vi "MotionProfileBegin.vi"(8 "error in (no error)":errorcluster) -> (0 "error out":errorcluster)   [LabVIEW 2019, in "Drive.lvlib" / "CTRE Drive.lvclass"]
uses:
  CTRE Drive.lvclass
  <vilib>/Rock Robotics/WPI/ThirdParty/Phoenix-LabVIEW/Motor Controller/Controls/CTRE_Phoenix_MotorControl_MotionProfileTrajectoryPoint.ctl
  <vilib>/Utility/file.llb/Read Delimited Spreadsheet (DBL).vi
  <vilib>/Rock Robotics/WPI/ThirdParty/Phoenix-LabVIEW/Motor Controller/Closed Loop/Motion Profile/CTRE_Phoenix_MotorControl_BufferedTrajectoryPointStream_WriteAll.vi
  <vilib>/Rock Robotics/WPI/ThirdParty/Phoenix-LabVIEW/Motor Controller/Closed Loop/Motion Profile/CTRE_Phoenix_MotorControl_BufferedTrajectoryPointStream_WriteOne.vi
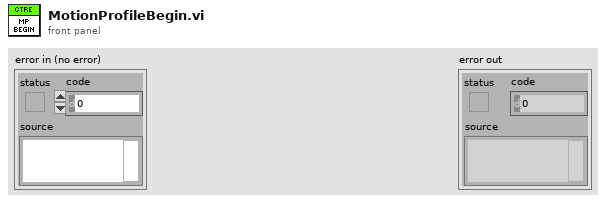
[diagram p1: front panel]
types:
  T1 = typedef "CTRE_Phoenix_MotorControl_MotionProfileTrajectoryPoint.ctl" = cluster{"Position":dbl, "Velocity":dbl, "Arbitrary Feed Forward":dbl, "Auxiliary Position":dbl, "Auxiliary Velocity":dbl, "Auxiliary Arbitrary Feed Forward":dbl, "Profile Slot Select":i32, "Auxiliary Profile Slot Select":i32, "isLastPoint?":bool, "Zero Position?":bool, "durationMs":u32, "Use Aux PID?":bool}
  T2 = typedef "CTRE_Phoenix_MotorControl_BufferedTrajectoryPointStream_DeviceRef.ctl" = cluster{"Handle":u64, "Library Path":path}
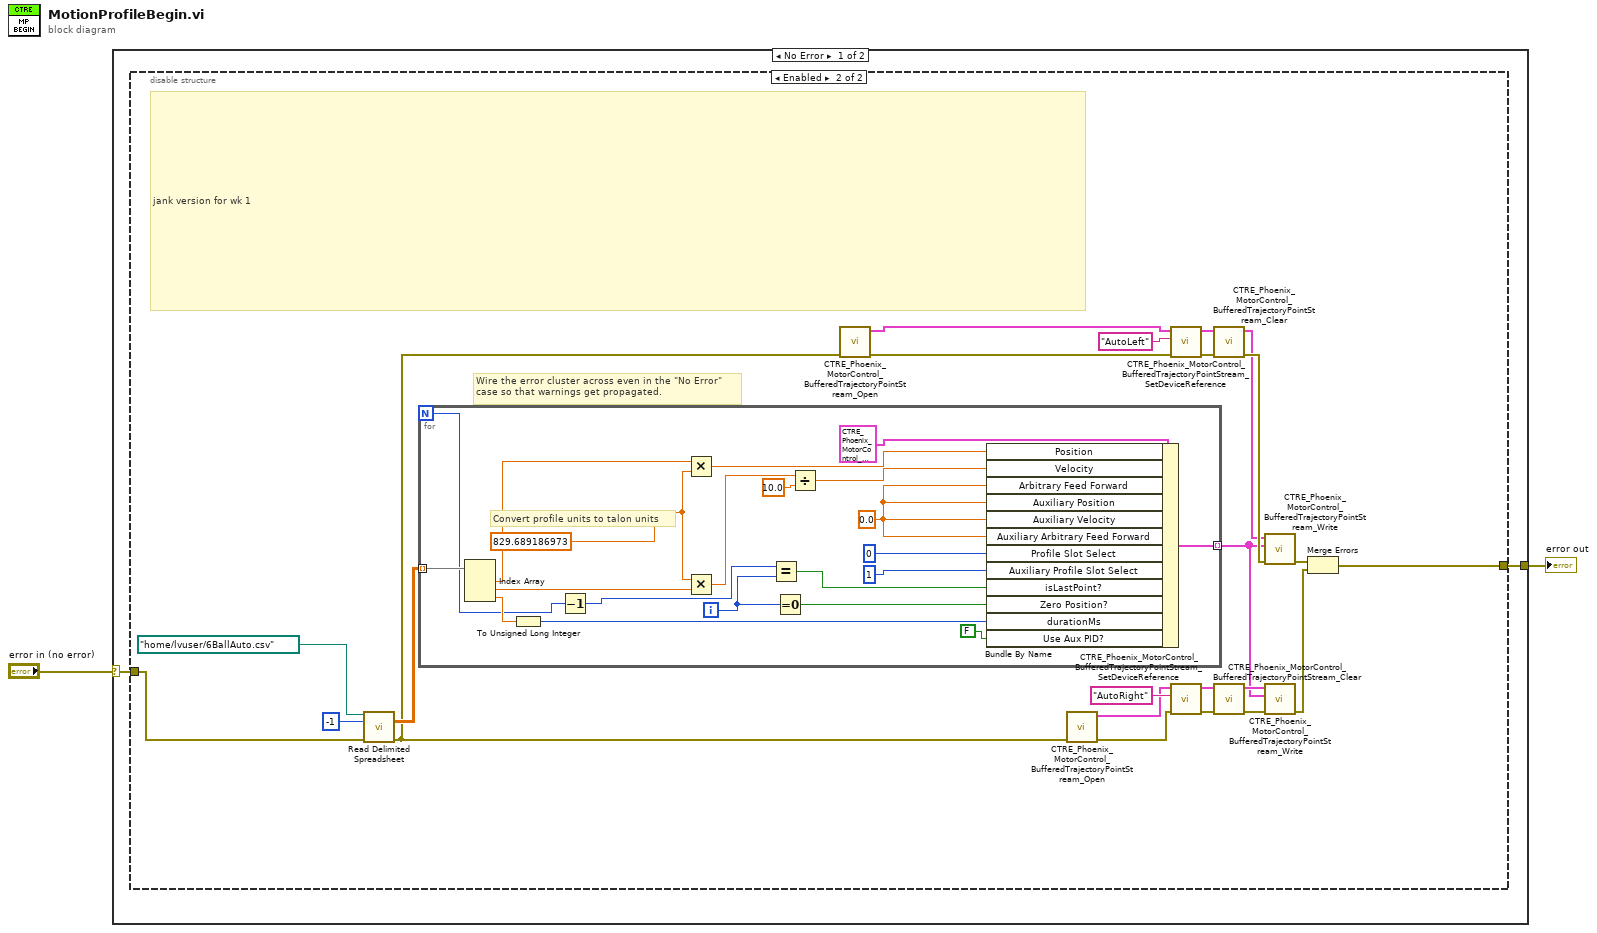
[diagram p0: block diagram]
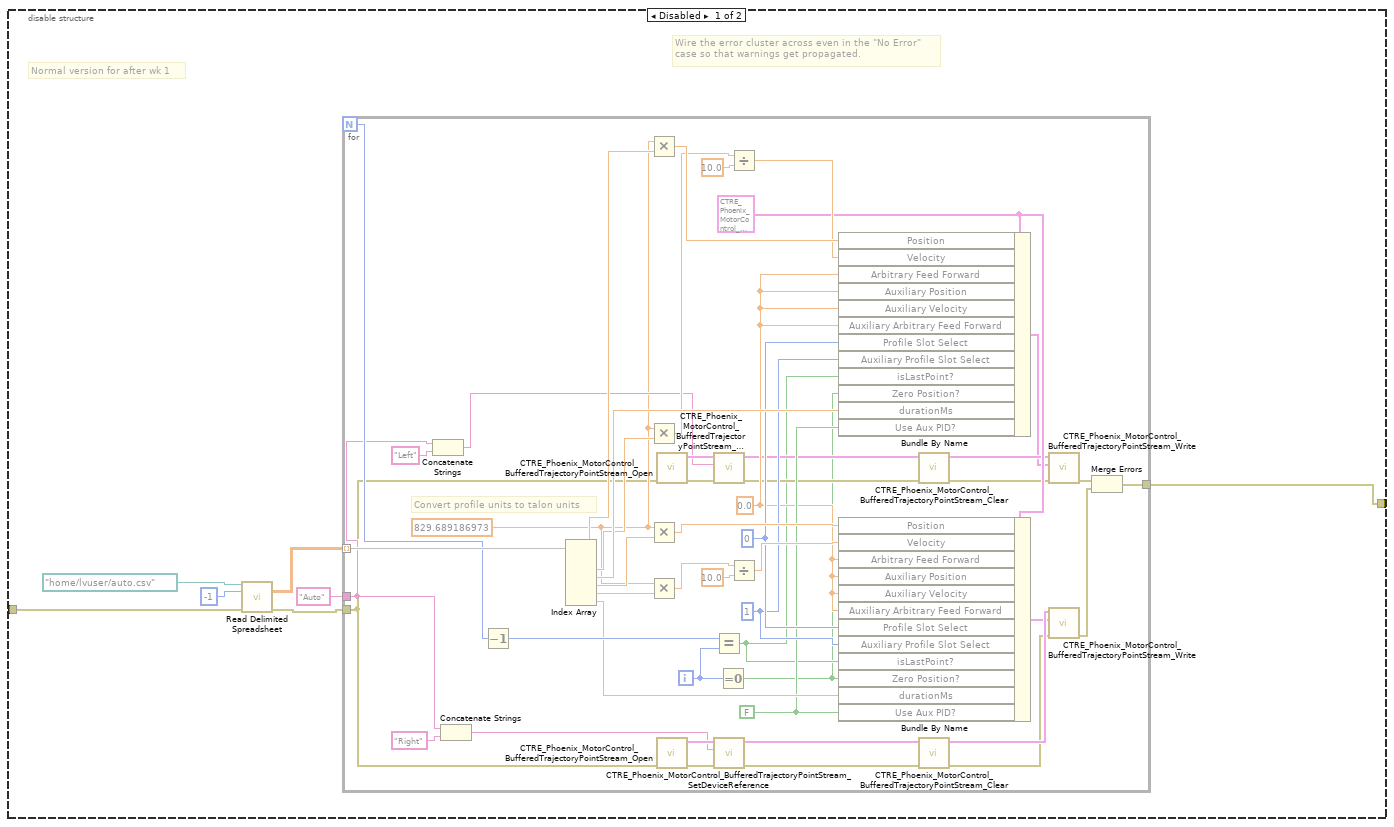
[diagram p2: hidden frame]
diagram:
  n1 = case shown="No Error" "error in (no error)" {
    selector: "error in (no error)" -> [w4 w105]
    tunnel: [w3 w105] -> w1
    frame No Error {
      n2 = disable-structure shown="Enabled" {
        disable-tunnel: w4 -> [w10 w80]
        disable-tunnel: [w9 w63] -> w3
        frame Disabled {
          # "Normal version for after wk 1"
          # "Wire the error cluster across even in the \"No Error\"\ncase so that warnings get propagated."
          n3 = call-poly <vilib>:"Read Delimited Spreadsheet.vi"("file path (dialog if empty)"=path "/home/lvuser/auto.csv" ("file path (use dialog)"), "number of rows (all:-1)"=-1, "error in (no error)"=w10) -> ("all rows"=w8:dbl[][], "error out"=w7:errorcluster)  [unwired: 7 in, 4 out]
          n4 = for {
            N -> [w42]
            tunnel: w8 -> [w52] mode=indexing
            tunnel: "Auto" -> [w30]
            tunnel: w7 -> [w15]
            tunnel: [w12] -> w9
            i -> [w38]
            w18 = 829.689186973 ("x")
            w41 = FALSE ("Use Aux PID?")
            w43 = 1 ("Auxiliary Profile Slot Select")
            w44 = 0 ("Profile Slot Select")
            w39 = 0.0 ("Arbitrary Feed Forward")
            w40 = T1 {"Position"=0.0, "Velocity"=0.0, "Arbitrary Feed Forward"=0.0, "Auxiliary Position"=0.0, "Auxiliary Velocity"=0.0, "Auxiliary Arbitrary Feed Forward"=0.0, "Profile Slot Select"=0, "Auxiliary Profile Slot Select"=0, "isLastPoint?"=FALSE, "Zero Position?"=FALSE, "durationMs"=0, "Use Aux PID?"=FALSE} ("Trajectory Point")
            # "Convert profile units to talon units"
            n5 = Concatenate Strings(w30, "Left" ("string")) -> (w28:string)
            n6 = Concatenate Strings(w30, "Right" ("string")) -> (w27:string)
            n7 = Decrement(x=w42) -> (x-1=w60:i32)
            n8 = Index Array(array=w52) -> (element #1=w58:dbl, element #2=w54:dbl, element #3=w59:dbl, element #4=w49:dbl, element #5=w48:dbl, element #6=w47:dbl)  [unwired: 6 in]
            n9 = Multiply(x=w18, y=w58) -> (x*y=w57:dbl)
            n10 = Multiply(x=w18, y=w54) -> (x*y=w56:dbl)
            n11 = Multiply(x=w18, y=w49) -> (x*y=w46:dbl)
            n12 = Multiply(x=w18, y=w48) -> (x*y=w51:dbl)
            n13 = call <vilib>:"CTRE_Phoenix_MotorControl_BufferedTrajectoryPointStream_Open.vi"("error in"=w15) -> ("error out"=w21:errorcluster, "BufferedTrajectoryPointStream_DevRef"=w32:T2)  [unwired: 9 in]
            n14 = call <vilib>:"CTRE_Phoenix_MotorControl_BufferedTrajectoryPointStream_Open.vi"("error in"=w15) -> ("error out"=w25:errorcluster, "BufferedTrajectoryPointStream_DevRef"=w35:T2)  [unwired: 9 in]
            n15 = call <vilib>:"CTRE_Phoenix_MotorControl_BufferedTrajectoryPointStream_SetDeviceReference.vi"("error in (no error)"=w21, "refnum name"=w28, "BufferedTrajectoryPointStream_DevRef"=w32) -> ("error out"=w22:errorcluster, "BufferedTrajectoryPointStream_DevRef"=w33:T2)  [unwired: 7 in]
            n16 = Equal?(x=w60, y=w38) -> (x = y?=w17:bool)
            n17 = call <vilib>:"CTRE_Phoenix_MotorControl_BufferedTrajectoryPointStream_SetDeviceReference.vi"("error in (no error)"=w25, "refnum name"=w27, "BufferedTrajectoryPointStream_DevRef"=w35) -> ("error out"=w26:errorcluster, "BufferedTrajectoryPointStream_DevRef"=w36:T2)  [unwired: 7 in]
            n18 = Equal To 0?(x=w38) -> (x = 0?=w16:bool)
            n19 = Divide(x=w56, y=10.0) -> (x/y=w53:dbl)
            n20 = Divide(x=w51, y=10.0) -> (x/y=w45:dbl)
            n21 = Bundle By Name(cluster=w40, "Position"=w57, "Velocity"=w53, "Arbitrary Feed Forward"=w39, "Auxiliary Position"=w39, "Auxiliary Velocity"=w39, "Auxiliary Arbitrary Feed Forward"=w39, "Profile Slot Select"=w44, "Auxiliary Profile Slot Select"=w43, "isLastPoint?"=w17, "Zero Position?"=w16, "durationMs"=w59, "Use Aux PID?"=w41) -> (w20:T1)
            n22 = Bundle By Name(cluster=w40, "Position"=w46, "Velocity"=w45, "Arbitrary Feed Forward"=w39, "Auxiliary Position"=w39, "Auxiliary Velocity"=w39, "Auxiliary Arbitrary Feed Forward"=w39, "Profile Slot Select"=w44, "Auxiliary Profile Slot Select"=w43, "isLastPoint?"=w17, "Zero Position?"=w16, "durationMs"=w47, "Use Aux PID?"=w41) -> (w19:T1)
            n23 = call <vilib>:"CTRE_Phoenix_MotorControl_BufferedTrajectoryPointStream_Clear.vi"("error in"=w22, "BufferedTrajectoryPointStream_DevRef"=w33) -> ("error out"=w23:errorcluster, "BufferedTrajectoryPointStream_DevRef"=w34:T2)  [unwired: 8 in]
            n24 = call <vilib>:"CTRE_Phoenix_MotorControl_BufferedTrajectoryPointStream_Clear.vi"("error in"=w26, "BufferedTrajectoryPointStream_DevRef"=w36) -> ("error out"=w24:errorcluster, "BufferedTrajectoryPointStream_DevRef"=w37:T2)  [unwired: 8 in]
            n25 = call-poly <vilib>:"CTRE_Phoenix_MotorControl_BufferedTrajectoryPointStream_Write.vi"("error in"=w23, "Trajectory Point"=w20, "BufferedTrajectoryPointStream_DevRef"=w34) -> ("error out"=w14:errorcluster)  [unwired: 7 in, 1 out]
            n26 = call-poly <vilib>:"CTRE_Phoenix_MotorControl_BufferedTrajectoryPointStream_Write.vi"("error in"=w24, "Trajectory Point"=w19, "BufferedTrajectoryPointStream_DevRef"=w37) -> ("error out"=w13:errorcluster)  [unwired: 7 in, 1 out]
            n27 = Merge Errors(w14, w13) -> (w12:errorcluster)
          }
        }
        frame Enabled {
          # "Wire the error cluster across even in the \"No Error\"\ncase so that warnings get propagated."
          # "jank version for wk 1"
          n28 = call-poly <vilib>:"Read Delimited Spreadsheet.vi"("file path (dialog if empty)"=path "/home/lvuser/6BallAuto.csv" ("file path (use dialog)"), "number of rows (all:-1)"=-1, "error in (no error)"=w80) -> ("all rows"=w82:dbl[][], "error out"=w64:errorcluster)  [unwired: 7 in, 4 out]
          n29 = for {
            N -> [w93]
            tunnel: w82 -> [w96] mode=indexing
            tunnel: [w85] -> w61 mode=indexing
            i -> [w89]
            w84 = 829.689186973 ("x")
            w90 = 0.0 ("Arbitrary Feed Forward")
            # "Convert profile units to talon units"
            n30 = Index Array(array=w96) -> (element #1=w102:dbl, element #2=w98:dbl, element #3=w103:dbl)  [unwired: 3 in]
            n31 = To Unsigned Long Integer(number=w103) -> (unsigned 32bit integer=w86:u32)
            n32 = Decrement(x=w93) -> (x-1=w104:i32)
            n33 = Multiply(x=w102, y=w84) -> (x*y=w101:dbl)
            n34 = Multiply(x=w84, y=w98) -> (x*y=w100:dbl)
            n35 = Equal?(x=w104, y=w89) -> (x = y?=w88:bool)
            n36 = Equal To 0?(x=w89) -> (x = 0?=w87:bool)
            n37 = Divide(x=w100, y=10.0) -> (x/y=w97:dbl)
            n38 = Bundle By Name(cluster=T1 {"Position"=0.0, "Velocity"=0.0, "Arbitrary Feed Forward"=0.0, "Auxiliary Position"=0.0, "Auxiliary Velocity"=0.0, "Auxiliary Arbitrary Feed Forward"=0.0, "Profile Slot Select"=0, "Auxiliary Profile Slot Select"=0, "isLastPoint?"=FALSE, "Zero Position?"=FALSE, "durationMs"=0, "Use Aux PID?"=FALSE} ("Trajectory Point"), "Position"=w101, "Velocity"=w97, "Arbitrary Feed Forward"=w90, "Auxiliary Position"=w90, "Auxiliary Velocity"=w90, "Auxiliary Arbitrary Feed Forward"=w90, "Profile Slot Select"=0, "Auxiliary Profile Slot Select"=1, "isLastPoint?"=w88, "Zero Position?"=w87, "durationMs"=w86, "Use Aux PID?"=FALSE) -> (w85:T1)
          }
          n39 = call <vilib>:"CTRE_Phoenix_MotorControl_BufferedTrajectoryPointStream_Open.vi"("error in"=w64) -> ("error out"=w79:errorcluster, "BufferedTrajectoryPointStream_DevRef"=w77:T2)  [unwired: 9 in]
          n40 = call <vilib>:"CTRE_Phoenix_MotorControl_BufferedTrajectoryPointStream_Open.vi"("error in"=w64) -> ("error out"=w71:errorcluster, "BufferedTrajectoryPointStream_DevRef"=w69:T2)  [unwired: 9 in]
          n41 = call <vilib>:"CTRE_Phoenix_MotorControl_BufferedTrajectoryPointStream_SetDeviceReference.vi"("error in (no error)"=w79, "refnum name"="AutoLeft", "BufferedTrajectoryPointStream_DevRef"=w77) -> ("error out"=w76:errorcluster, "BufferedTrajectoryPointStream_DevRef"=w75:T2)  [unwired: 7 in]
          n42 = call <vilib>:"CTRE_Phoenix_MotorControl_BufferedTrajectoryPointStream_SetDeviceReference.vi"("error in (no error)"=w71, "refnum name"="AutoRight", "BufferedTrajectoryPointStream_DevRef"=w69) -> ("error out"=w68:errorcluster, "BufferedTrajectoryPointStream_DevRef"=w67:T2)  [unwired: 7 in]
          n43 = call <vilib>:"CTRE_Phoenix_MotorControl_BufferedTrajectoryPointStream_Clear.vi"("error in"=w76, "BufferedTrajectoryPointStream_DevRef"=w75) -> ("error out"=w74:errorcluster, "BufferedTrajectoryPointStream_DevRef"=w73:T2)  [unwired: 8 in]
          n44 = call <vilib>:"CTRE_Phoenix_MotorControl_BufferedTrajectoryPointStream_Clear.vi"("error in"=w68, "BufferedTrajectoryPointStream_DevRef"=w67) -> ("error out"=w66:errorcluster, "BufferedTrajectoryPointStream_DevRef"=w65:T2)  [unwired: 8 in]
          n45 = call-poly <vilib>:"CTRE_Phoenix_MotorControl_BufferedTrajectoryPointStream_Write.vi"("error in"=w74, "Motion Profile Trajectory Point Array"=w61, "BufferedTrajectoryPointStream_DevRef"=w73) -> ("error out"=w72:errorcluster)  [unwired: 7 in, 1 out]
          n46 = call-poly <vilib>:"CTRE_Phoenix_MotorControl_BufferedTrajectoryPointStream_Write.vi"("error in"=w66, "Motion Profile Trajectory Point Array"=w61, "BufferedTrajectoryPointStream_DevRef"=w65) -> ("error out"=w62:errorcluster)  [unwired: 7 in, 1 out]
          n47 = Merge Errors(w72, w62) -> (w63:errorcluster)
        }
      }
    }
    frame Error {
    }
  }
  "error out" <- w1
